vi "my_PICO_Run.vi"(6 "布尔输入":bool, 7 "stop":bool, 8 "簇 3":T2, 9 "簇 4":T2, 10 "n_tbase(default)":u32, 11 "n_samp(default)":u64) -> (0 "MultiBuffers (Max or non-aggregated)":T1(array[cluster]), 1 "MultiBuffers (Max or non-aggregated) 2":T1(array[cluster]), 2 "簇 2":T4, 3 "簇":T4, 5 "布尔输出":bool)   [LabVIEW 2024]
uses:
  shared/PicoBuffers.ctl
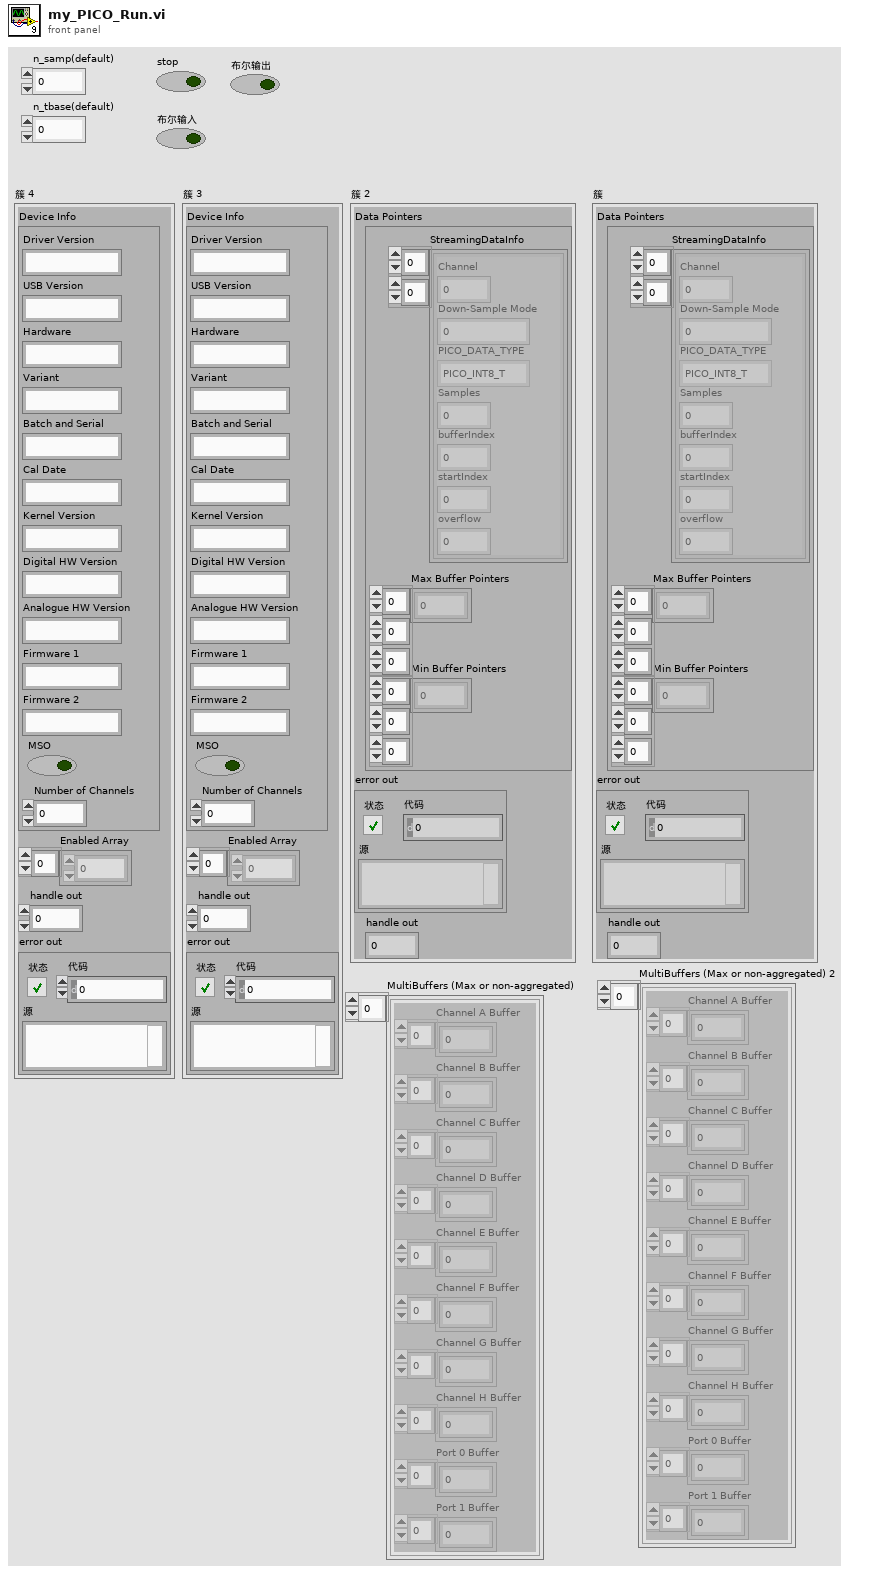
[diagram p1: front panel]
types:
  T1 = cluster{"Channel A Buffer":i16[], "Channel B Buffer":i16[], "Channel C Buffer":i16[], "Channel D Buffer":i16[], "Channel E Buffer":i16[], "Channel F Buffer":i16[], "Channel G Buffer":i16[], "Channel H Buffer":i16[], "Port 0 Buffer":i16[], "Port 1 Buffer":i16[]}[]
  T2 = cluster{"Device Info":cluster{"Driver Version":string, "USB Version":string, "Hardware":string, "Variant":string, "Batch and Serial":string, "Cal Date":string, "Kernel Version":string, "Digital HW Version":string, "Analogue HW Version":string, "Firmware 1":string, "Firmware 2":string, "MSO":bool, "Number of Channels":i16}, "Enabled Array":i16[], "handle out":i16, "error out":errorcluster}
  T3 = typedef "PicoBuffers.ctl" = cluster{"Max Buffer Pointers":u64[][][], "Min Buffer Pointers":u64[][][], "StreamingDataInfo":cluster{"Channel":u32, "Down-Sample Mode":u32, "PICO_DATA_TYPE":enum32{"PICO_INT8_T", "PICO_INT16_T", "PICO_INT32_T", "PICO_UINT32_T", "PICO_INT64_T", ""}, "Samples":i32, "bufferIndex":u64, "startIndex":i32, "overflow":i16}[][]}
  T4 = cluster{"Data Pointers":T3, "error out":errorcluster, "handle out":i16}
  T5 = cluster{"Driver Version":string, "USB Version":string, "Hardware":string, "Variant":string, "Batch and Serial":string, "Cal Date":string, "Kernel Version":string, "Digital HW Version":string, "Analogue HW Version":string, "Firmware 1":string, "Firmware 2":string, "MSO":bool, "Number of Channels":i16}
  T6 = cluster{u64, "n_samp(default)":u64, "n_tbase(default)":u32}
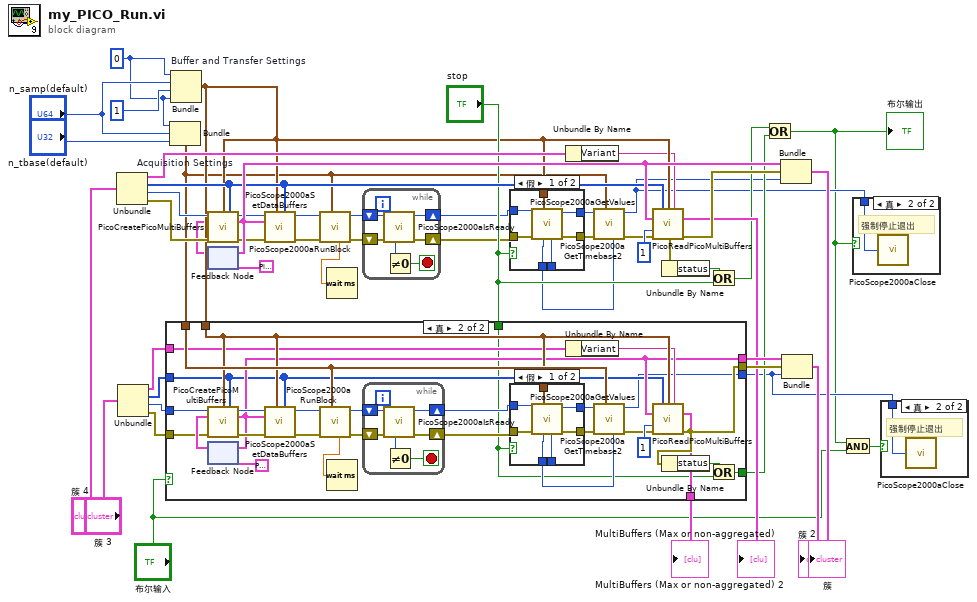
[diagram p0: block diagram]
diagram:
  w23 = u64 0
  n1 = Unbundle("簇 4") -> ("Device Info"=w38:T5, "Enabled Array"=w37:i16[], "handle out"=w36:i16, "error out"=w35:errorcluster)
  n2 = Unbundle("簇 3") -> ("Device Info"=w43:T5, "Enabled Array"=w42:i16[], "handle out"=w41:i16, "error out"=w40:errorcluster)
  n3 = Bundle "Acquisition Settings"(w23, "n_samp(default)"="n_samp(default)", "n_tbase(default)"="n_tbase(default)") -> (w25:T6)  [unwired: 1 in]
  n4 = Bundle "Buffer and Transfer Settings"(w23, "n_samp(default)"="n_samp(default)", u64 1, w23) -> (w26:cluster{u64, "n_samp(default)":u64, u64, u64})  [unwired: 1 in]
  n5 = case shown="真" "布尔输入" {
    tunnel: w25 -> [_ w78]
    tunnel: w26 -> [_ w77]
    tunnel: [_ w76] -> w28
    tunnel: w43 -> [_ w58]
    tunnel: w40 -> [_ w57]
    tunnel: w41 -> [_ w56]
    tunnel: [_ w55] -> w45
    tunnel: w42 -> [_ w54]
    tunnel: [_ w53] -> w46
    tunnel: [_ w52] -> w4
    tunnel: [_ w51] -> w31
    tunnel: "stop" -> [_ w50]
    frame False {
    }
    frame True {
      n6 = feedback #1(T3 {"Max Buffer Pointers"=[], "Min Buffer Pointers"=[], "StreamingDataInfo"=[]} ("Data Pointers")) -> (w74:T3)
      n7 = call "PicoCreatePicoMultiBuffers.vi"("Buffer and Transfer Settings"=w77, "enabled array"=w54, "Data Pointers In"=w74, "error in (no error)"=w57) -> ("Data Pointers"=w55:T3, "error out"=w73:errorcluster)  [unwired: 10 in]
      n8 = feedback-in #1(w55) -> ()
      n9 = call "PicoScope2000aSetDataBuffers.vi"("enabled array"=w54, "Buffer and Transfer Settings"=w77, "error in (no error)"=w73, "Data Pointers In"=w55, "handle in"=w56) -> ("error out"=w71:errorcluster, "handle out"=w72:i16)  [unwired: 5 in]
      n10 = call "PicoScope2000aRunBlock.vi"("Acquisition Settings"=w78, "error in (no error)"=w71, "handle in"=w72) -> ("error out"=w60:errorcluster, "handle out"=w61:i16, "timeIndisposedMs"=w66:dbl)  [unwired: 5 in, 1 out]
      n11 = Wait (ms)(milliseconds to wait=w66) -> ()  [unwired: 1 out]
      n12 = while {
        shift-right: [w92] -> w64
        shift-left: w60 -> [w93]
        shift-right: [w91] -> w63
        shift-left: w61 -> [w90]
        stop <- w88 stop-if-true
        n13 = call "PicoScope2000aIsReady.vi"("error in (no error)"=w93, "handle in"=w90) -> ("error out"=w92:errorcluster, "handle out"=w91:i16, "ready"=w89:i16)  [unwired: 7 in]
        n14 = Not Equal To 0?(x=w89) -> (x != 0?=w88:bool)
      }
      n15 = case shown="假" w50 {
        tunnel: w64 -> [w85 w86]
        tunnel: w63 -> [w84 w87]
        tunnel: [w83 w87] -> w68
        tunnel: [w82 w86] -> w67
        tunnel: w77 -> [w81 _]
        tunnel: [w80 _] -> _
        tunnel: [w79 _] -> w65
        frame False {
          n16 = call "PicoScope2000aGetValues.vi"("Buffer and Transfer Settings"=w81, "error in (no error)"=w85, "handle in"=w84) -> ("error out"=w82:errorcluster, "handle out"=w83:i16, "overflow"=w80:i16, "noOfSamples"=w79:u64)  [unwired: 5 in]
        }
        frame True {
        }
      }
      n17 = Unbundle By Name(w58) -> ("Variant"=w62:string)
      n18 = call "PicoScope2000aGetTimebase2.vi"("Number of Samples"=w65, "Acquisition Settings"=w78, "error in (no error)"=w67, "handle in"=w68) -> ("error out"=w69:errorcluster, "handle out"=w52:i16)  [unwired: 5 in, 1 out]
      n19 = call "PicoReadPicoMultiBuffers.vi"("enabled array"=w54, "Buffer and Transfer Settings"=w77, "Variant"=w62, "Data Pointers"=w55, "No of Buffers"=1, "error in (no error)"=w69) -> ("MultiBuffers (Max or non-aggregated)"=w51:T1, "error out"=w53:errorcluster)  [unwired: 7 in, 1 out]
      n20 = Unbundle By Name(w53) -> ("status"=w59:bool)
      n21 = Or(x=w59, y=w50) -> (x .or. y?=w76:bool)
    }
  }
  "MultiBuffers (Max or non-aggregated) 2" <- w31
  n22 = feedback #2(T3 {"Max Buffer Pointers"=[], "Min Buffer Pointers"=[], "StreamingDataInfo"=[]} ("Data Pointers")) -> (w21:T3)
  n23 = call "PicoCreatePicoMultiBuffers.vi"("Buffer and Transfer Settings"=w26, "enabled array"=w37, "Data Pointers In"=w21, "error in (no error)"=w35) -> ("Data Pointers"=w44:T3, "error out"=w20:errorcluster)  [unwired: 10 in]
  n24 = feedback-in #2(w44) -> ()
  n25 = call "PicoScope2000aSetDataBuffers.vi"("enabled array"=w37, "Buffer and Transfer Settings"=w26, "error in (no error)"=w20, "Data Pointers In"=w44, "handle in"=w36) -> ("error out"=w18:errorcluster, "handle out"=w19:i16)  [unwired: 5 in]
  n26 = call "PicoScope2000aRunBlock.vi"("Acquisition Settings"=w25, "error in (no error)"=w18, "handle in"=w19) -> ("error out"=w7:errorcluster, "handle out"=w8:i16, "timeIndisposedMs"=w13:dbl)  [unwired: 5 in, 1 out]
  n27 = Wait (ms)(milliseconds to wait=w13) -> ()  [unwired: 1 out]
  n28 = while {
    shift-right: [w98] -> w11
    shift-left: w7 -> [w99]
    shift-right: [w97] -> w10
    shift-left: w8 -> [w96]
    stop <- w94 stop-if-true
    n29 = call "PicoScope2000aIsReady.vi"("error in (no error)"=w99, "handle in"=w96) -> ("error out"=w98:errorcluster, "handle out"=w97:i16, "ready"=w95:i16)  [unwired: 7 in]
    n30 = Not Equal To 0?(x=w95) -> (x != 0?=w94:bool)
  }
  n31 = case shown="假" "stop" {
    tunnel: w11 -> [w106 w107]
    tunnel: w10 -> [w105 w108]
    tunnel: [w104 w108] -> w15
    tunnel: [w103 w107] -> w14
    tunnel: w26 -> [w102 _]
    tunnel: [w101 _] -> _
    tunnel: [w100 _] -> w12
    frame False {
      n32 = call "PicoScope2000aGetValues.vi"("Buffer and Transfer Settings"=w102, "error in (no error)"=w106, "handle in"=w105) -> ("error out"=w103:errorcluster, "handle out"=w104:i16, "overflow"=w101:i16, "noOfSamples"=w100:u64)  [unwired: 5 in]
    }
    frame True {
    }
  }
  n33 = Unbundle By Name(w38) -> ("Variant"=w9:string)
  n34 = call "PicoScope2000aGetTimebase2.vi"("Number of Samples"=w12, "Acquisition Settings"=w25, "error in (no error)"=w14, "handle in"=w15) -> ("error out"=w16:errorcluster, "handle out"=w5:i16)  [unwired: 5 in, 1 out]
  n35 = call "PicoReadPicoMultiBuffers.vi"("enabled array"=w37, "Buffer and Transfer Settings"=w26, "Variant"=w9, "Data Pointers"=w44, "No of Buffers"=1, "error in (no error)"=w16) -> ("MultiBuffers (Max or non-aggregated)"=→"MultiBuffers (Max or non-aggregated)":T1, "error out"=w49:errorcluster)  [unwired: 7 in, 1 out]
  n36 = Unbundle By Name(w49) -> ("status"=w6:bool)
  n37 = Or(x=w6, y="stop") -> (x .or. y?=w27:bool)
  n38 = Or(x=w27, y=w28) -> (x .or. y?=w1:bool)
  "布尔输出" <- w1
  n39 = Bundle("Data Pointers"=w44, "error out"=w49, "handle out"=w5) -> (→"簇":T4)  [unwired: 1 in]
  n40 = Bundle("Data Pointers"=w45, "error out"=w46, "handle out"=w4) -> (→"簇 2":T4)  [unwired: 1 in]
  n41 = And(x=w1, y="布尔输入") -> (x .and. y?=w3:bool)
  n42 = case shown="真" w1 {
    tunnel: w5 -> [_ w109]
    frame False {
    }
    frame True {
      # "强制停止退出"
      n43 = call "PicoScope2000aClose.vi"("handle"=w109) -> ()
    }
  }
  n44 = case shown="真" w3 {
    tunnel: w4 -> [_ w110]
    frame False {
    }
    frame True {
      # "强制停止退出"
      n45 = call "PicoScope2000aClose.vi"("handle"=w110) -> ()
    }
  }
